vi "NewFITSHead.vi"(0 "file path":path, 1 "FITS":T1={"BITPIX"=8.0, "NAXIS"=2.0, "NAXIS1"=100.0, "NAXIS2"=100.0, "NAXIS3"=100.0, "BZERO"=0.0, "BSCALE"=1.0}, 2 "error in":errorcluster) -> (3 "FITS file":T2, 5 "offset":u32, 6 "error out":errorcluster)   [LabVIEW 2011]
panel:
  out "length":i32
  # "bits per pixel\n?\nY\nX\nPlanes\noffset0\nSclae1"
  # "Hedaer is 36x80Bytes Ascii\nBitte mit SIMPLE = T und END"
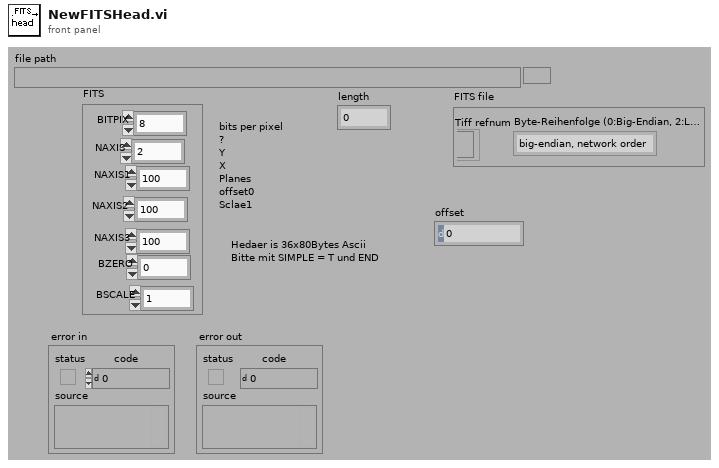
[diagram p1: front panel]
types:
  T1 = cluster{"BITPIX":sgl, "NAXIS":sgl, "NAXIS1":sgl, "NAXIS2":sgl, "NAXIS3":sgl, "BZERO":sgl, "BSCALE":sgl}
  T2 = cluster{"Tiff refnum":refnum<file>, "Byte-Reihenfolge (0:Big-Endian, 2:LSB)":enum16{"big-endian, network order", "native, host order", "little-endian"}}
  T3 = enum16{"big-endian, network order", "native, host order", "little-endian"}
  T4 = enum16{"open", "replace", "create", "open or create", "replace or create", "replace or create with confirmation"}
  T5 = cluster{"refnum out":refnum<file>, "byte order (0:big-endian, network order)":enum16{"big-endian, network order", "native, host order", "little-endian"}}
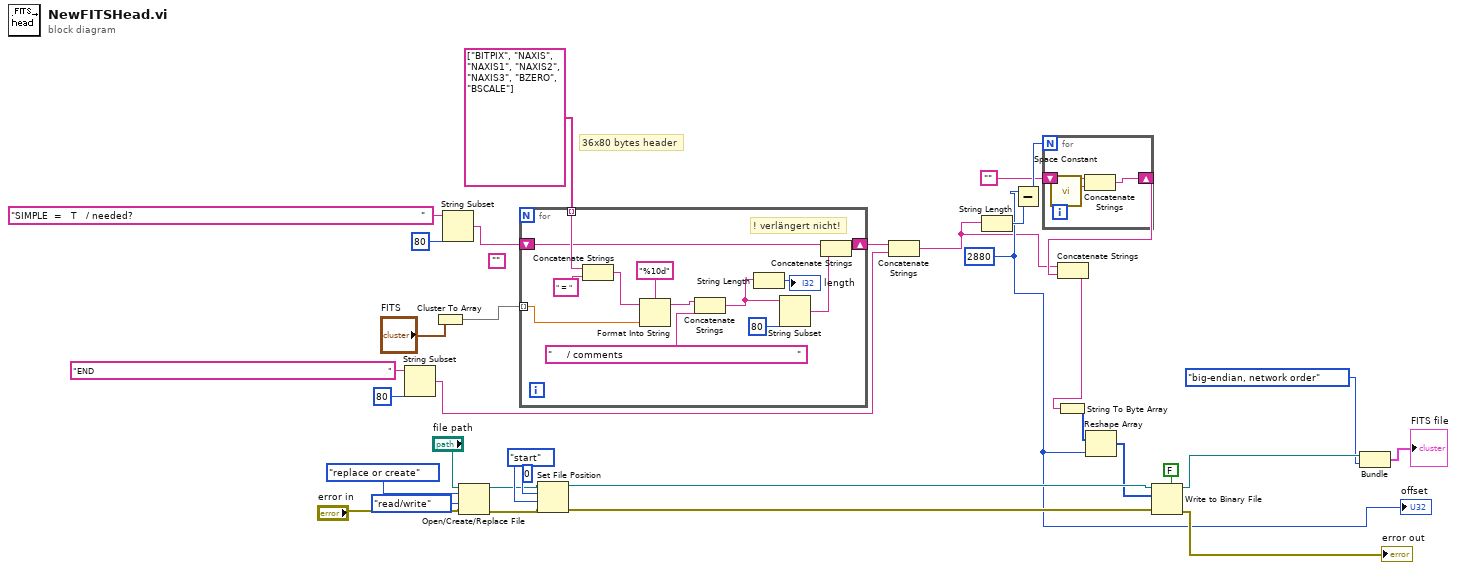
[diagram p0: block diagram]
diagram:
  w8 = 2880 ("dimension size")
  (unwired) ""
  # "36x80 bytes header"
  n1 = String Subset(string="END                                                                                                  ", length (rest)=80 ("length (rest)")) -> (substring=w1:string)  [unwired: 1 in]
  n2 = Cluster To Array(cluster="FITS") -> (array=w22:sgl[])
  n3 = String Subset(string="SIMPLE  =   T   / needed?                                                                                                ", length (rest)=80 ("length (rest)")) -> (substring=w5:string)  [unwired: 1 in]
  n4 = Open/Create/Replace File(file path (use dialog)="file path", error in="error in", operation (0:open)=T4."replace or create" ("Operation (0:Öffnen)"), access (0:read/write)=enum16{"read/write", "read-only", "write-only"}."read/write" ("Zugriff (0:Lesen/Schreiben)")) -> (refnum out=w25:refnum<file>, error out=w24:errorcluster)  [unwired: 3 out]
  n5 = for {
    tunnel: w22 -> [w47] mode=indexing
    shift-right: [w35] -> w12
    shift-left: w5 -> [w37]
    tunnel: string[] ["BITPIX", "NAXIS", "NAXIS1", "NAXIS2", "NAXIS3", "BZERO", "BSCALE"] -> [w45] mode=indexing
    # "! verlängert nicht!"
    n6 = Concatenate Strings(w45, " = " ("string")) -> (w43:string)
    n7 = Format Into String(format string="%10d", initial string=w43, w47) -> (resulting string=w42:string)  [unwired: 1 in, 1 out]
    n8 = Concatenate Strings(w42, "     / comments                                                          ") -> (w39:string)
    n9 = String Length(string=w39) -> (length=→"length":i32)
    n10 = String Subset(string=w39, length (rest)=80 ("length (rest)")) -> (substring=w36:string)  [unwired: 1 in]
    n11 = Concatenate Strings(w37, w36) -> (w35:string)
  }
  n12 = Set File Position(offset (in bytes) (0)=0 ("IFDoffset"), refnum=w25, from (0:start)=enum16{"start", "end", "current"}."start" ("pos mode (0:2)"), error in=w24) -> (refnum out=w27:refnum<file>, error out=w26:errorcluster)
  n13 = Concatenate Strings(w12, w1) -> (w2:string)
  n14 = String Length(string=w2) -> (length=w9:i32)
  n15 = Subtract(x=w8, y=w9) -> (x-y=w14:i32)
  n16 = for {
    N: w14 -> [_]
    shift-right: [w49] -> w11
    shift-left: "" -> [w48]
    n17 = call <vilib>:"Space Constant.vi"() -> ("String"=w50:string)
    n18 = Concatenate Strings(w48, w50) -> (w49:string)
  }
  n19 = Concatenate Strings(w2, w11) -> (w10:string)
  n20 = String To Byte Array(string=w10) -> (unsigned byte array=w20:u8[])
  n21 = Reshape Array(w20, w8) -> (w19:u8[])
  n22 = Write to Binary File(file (use dialog)=w27, data=w19, error in=w26, 5:FALSE ("Array- oder Stringgröße voranstellen? (T)")) -> (refnum out=w18:refnum<file>, error out=→"error out":errorcluster)  [unwired: 1 in, 2 out]
  n23 = Bundle("refnum out"=w18, "byte order (0:big-endian, network order)"=T3."big-endian, network order") -> (→"FITS file":T5)  [unwired: 1 out]
  "offset" <- w8
